vi "Configure Multi Eval Meas Trigger.vi"(4 "Minimum Trigger Gap (500e-6)":dbl=0.0005 format="%^.3e", 5 "Trigger Delay (0.0)":dbl format="%^.3e", 6 "Trigger Threshold (-20.0)":dbl=-20.0 format="%^.3e", 7 "Trigger Slope (Rising edge)":i32(ring) items=["Rising edge", "Falling Edge"], 8 "error in (no error)":errorcluster, 9 "Trigger Source (\"IF Power\")":string="IF Power", 10 "Instance (1)":T1=1, 11 "VISA resource name":refnum<visa-resource-name>) -> (0 "error out":errorcluster, 3 "VISA resource name out":refnum<visa-resource-name>)   [LabVIEW 2015, in "Rohde&Schwarz CMXP NR FR2 Measurement.lvlib"]
doc: "Configures multi evaluation measurement trigger subsystem.\n\nAttributes:\nRSCMXPNRFR2M_ATTR_MULTI_EVAL_MEASUREMENT_TRIGGER_SOURCE\nRSCMXPNRFR2M_ATTR_MULTI_EVAL_MEASUREMENT_TRIGGER_SLOPE\nRSCMXPNRFR2M_ATTR_MULTI_EVAL_MEASUREMENT_TRIGGER_THRESHOLD\nRSCMXPNRFR2M_ATTR_MULTI_EVAL_MEASUREMENT_TRIGGER_DELAY\nRSCMXPNRFR2M_ATTR_MULTI_EVAL_MEASUREMENT_MINIMUM_TRIGGER_GAP\n\nRemote-control commands:\nTRIGger:NRMMw:MEAS<i>:MEValuation:SOURce\nTRIGger:NRMMw:MEAS<i>:MEValuation:SLOPe\nTRIGger:NRMMw:MEAS<i>:MEValuation:THReshold\nTRIGger:NRMMw:MEAS<i>:MEValuation:DELay\nTRIGger:NRMMw:MEAS<i>:MEValuation:MGAP"
uses:
  <instrlib>/Rohde&Schwarz CMXP NR FR2 Measurement/Rohde&Schwarz CMXP NR FR2 Measurement.lvlib
  <instrlib>/Rohde&Schwarz CMXP NR FR2 Measurement/Private/_Instance.ctl
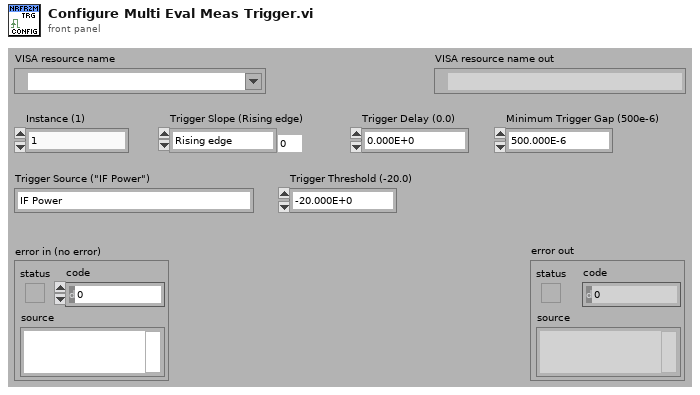
[diagram p1: front panel]
types:
  T1 = typedef "Rohde&Schwarz CMXP NR FR2 Measurement.lvlib/_Instance.ctl" = i32
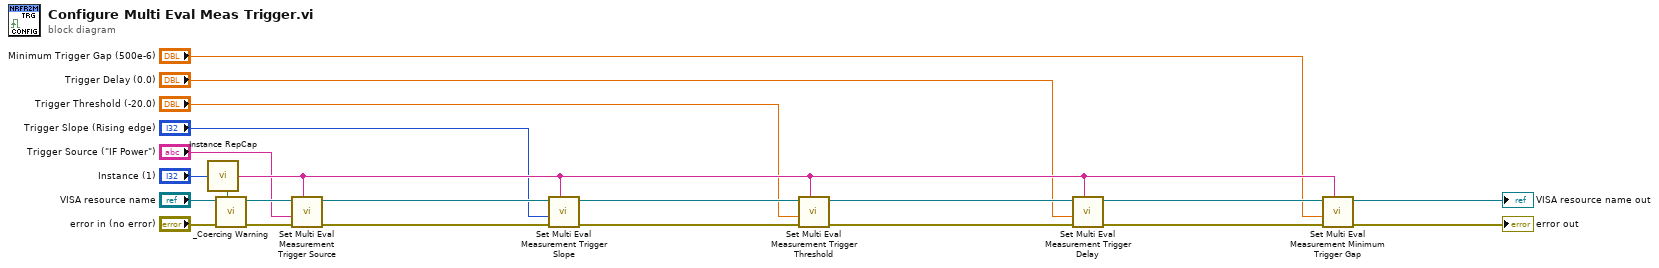
[diagram p0: block diagram]
diagram:
  n1 = call <instrlib>:"Instance RepCap.vi"("Instance In"="Instance (1)") -> ("In Range?"=w10:bool, "RepCap Identifier Out"=w7:string)  [unwired: 1 in]
  n2 = call <instrlib>:"_Coercing Warning.vi"("In Range?"=w10, "error in (no error)"="error in (no error)", "VISA resource name"="VISA resource name") -> ("error out"=w8:errorcluster, "VISA resource name out"=w9:refnum<visa-resource-name>)  [unwired: 7 in]
  n3 = call "Set Multi Eval Measurement Trigger Source"("Repeated Capabilities"=w7, "error in (no error)"=w8, "Multi Eval Measurement Trigger Source ()"="Trigger Source (\"IF Power\")", "instrument handle"=w9) -> ("error out"=w21:errorcluster, "instrument handle out"=w22:refnum<visa-resource-name>)  [unwired: 6 in]
  n4 = call "Set Multi Eval Measurement Trigger Slope"("Repeated Capabilities"=w7, "error in (no error)"=w21, "Multi Eval Measurement Trigger Slope (0 - Rising edge)"="Trigger Slope (Rising edge)", "instrument handle"=w22) -> ("error out"=w19:errorcluster, "instrument handle out"=w20:refnum<visa-resource-name>)  [unwired: 6 in]
  n5 = call "Set Multi Eval Measurement Trigger Threshold"("Repeated Capabilities"=w7, "error in (no error)"=w19, "Multi Eval Measurement Trigger Threshold (0.0)"="Trigger Threshold (-20.0)", "instrument handle"=w20) -> ("error out"=w17:errorcluster, "instrument handle out"=w18:refnum<visa-resource-name>)  [unwired: 6 in]
  n6 = call "Set Multi Eval Measurement Trigger Delay"("Repeated Capabilities"=w7, "error in (no error)"=w17, "Multi Eval Measurement Trigger Delay (0.0)"="Trigger Delay (0.0)", "instrument handle"=w18) -> ("error out"=w13:errorcluster, "instrument handle out"=w14:refnum<visa-resource-name>)  [unwired: 6 in]
  n7 = call "Set Multi Eval Measurement Minimum Trigger Gap"("Repeated Capabilities"=w7, "error in (no error)"=w13, "Multi Eval Measurement Minimum Trigger Gap (0.0)"="Minimum Trigger Gap (500e-6)", "instrument handle"=w14) -> ("error out"=→"error out":errorcluster, "instrument handle out"=→"VISA resource name out":refnum<visa-resource-name>)  [unwired: 6 in]
